vi "interface initialization.vi"(11 "VI in":refnum<vi>) -> (0 "error out":errorcluster)   [LabVIEW 2018]
uses:
  <vilib>/Utility/miscctls.llb/LVPointTypeDef.ctl
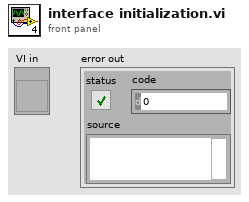
[diagram p1: front panel]
types:
  T1 = typedef "LVPointTypeDef.ctl" = cluster{"Horizontal":i16, "Vertical":i16}
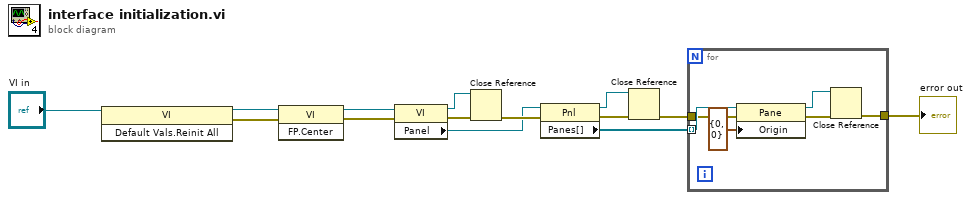
[diagram p0: block diagram]
diagram:
  n1 = invoke class="VI" method="Default Vals.Reinit All"(reference="VI in") -> (reference out=w4:refnum<vi>, error out=w3:errorcluster)  [unwired: 2 in, 1 out]
  n2 = invoke class="VI" method="FP.Center"(reference=w4, error in=w3) -> (reference out=w1:refnum<vi>, error out=w2:errorcluster)  [unwired: 1 in, 1 out]
  n3 = property class="VI"(reference=w1, error in=w2) -> (reference out=w11:refnum<vi>, error out=w12:errorcluster, "Panel"=w9:refnum<vi>)
  n4 = Close Reference(reference=w11, error in (no error)=w12) -> (error out=w10:errorcluster)
  n5 = property class="Pnl"(reference=w9, error in=w10) -> (reference out=w7:refnum<vi>, error out=w8:errorcluster, "Panes[]"=w6:refnum<vi>[])
  n6 = Close Reference(reference=w7, error in (no error)=w8) -> (error out=w5:errorcluster)
  n7 = for {
    tunnel: w6 -> [w20] mode=indexing
    tunnel: w5 -> [w19]
    tunnel: [w15] -> w14
    n8 = property class="Pane"(reference=w20, error in=w19, "Origin"=T1 {"Horizontal"=0, "Vertical"=0}) -> (reference out=w16:refnum<vi>, error out=w17:errorcluster)
    n9 = Close Reference(reference=w16, error in (no error)=w17) -> (error out=w15:errorcluster)
  }
  "error out" <- w14
